vi "Spy Flush Last Warning.vi"(8 "error in (no error)":errorcluster, 11 "Mock Error Handler In":refnum<class "Mock Error Handler.lvclass">) -> (0 "error out":errorcluster, 1 "Error":errorcluster, 3 "Mock Error Handler Out":refnum<class "Mock Error Handler.lvclass">)   [LabVIEW 2020, in "Mock Error Handler.lvclass"]
doc: "Spys on errors sent to the error handler. This Method requires a lock on the execution thread to prevent race conditions when testing other processes using the error handler."
uses:
  Mock Error Handler.lvclass
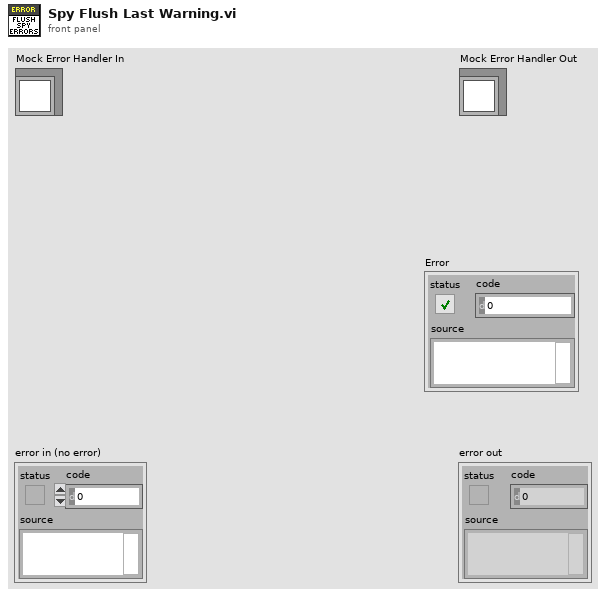
[diagram p1: front panel]
types:
  T1 = typedef "Mock Error Handler.lvclass/Error Message Data.ctl" = cluster{"Location":string, "Error":errorcluster}
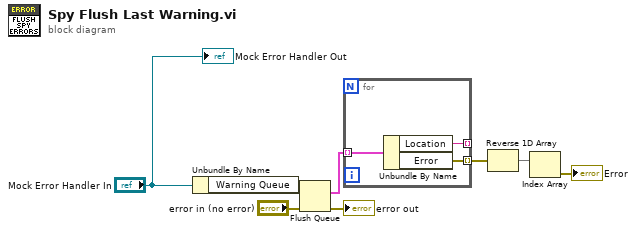
[diagram p0: block diagram]
diagram:
  n1 = Unbundle By Name("Mock Error Handler In") -> ("Warning Queue"=w1:refnum<queue>)
  n2 = Flush Queue(queue=w1, error in (no error)="error in (no error)") -> (remaining elements=w2:T1[], error out=→"error out":errorcluster)  [unwired: 1 out]
  n3 = for {
    tunnel: w2 -> [w11] mode=indexing
    tunnel: [w10] -> _ mode=indexing
    tunnel: [w9] -> w3 mode=indexing
    n4 = Unbundle By Name(w11) -> ("Location"=w10:string, "Error"=w9:errorcluster)
  }
  n5 = Reverse 1D Array(array=w3) -> (reversed array=w5:errorcluster[])
  n6 = Index Array(array=w5) -> (element=→"Error":errorcluster)  [unwired: 1 in]
  "Mock Error Handler Out" <- "Mock Error Handler In"
